vi "test_event.vi"() -> ()   [LabVIEW 2014]
panel:
  in  "Boolean 3":bool=TRUE
  out "Boolean 2":bool=TRUE
  out "Boolean":bool=TRUE
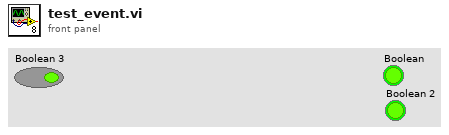
[diagram p1: front panel]
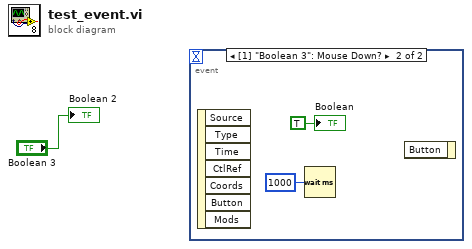
[diagram p0: block diagram]
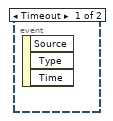
[diagram p2: hidden frame]
diagram:
  n1 = event shown="[1] \"Boolean 3\": Mouse Down?" {
    selector: _ -> [_ _]
    dyn-events: _ -> [_ _]
    timeout: _ -> [_ _]
    event Timeout {
      n2 = event-data() -> ()  [unwired: 1 in, 3 out]
    }
    event "Boolean 3": Mouse Down? {
      n3 = event-data() -> ()  [unwired: 1 in, 7 out]
      n4 = Wait (ms)(milliseconds to wait=u32 1000) -> ()  [unwired: 1 out]
      n5 = event-data() -> ()  [unwired: 2 in, 1 out]
      "Boolean" <- TRUE ("Boolean")
    }
  }
  "Boolean 2" <- "Boolean 3"
